vi "find nearest neighbors index float.vi"(0 "index_id":u64, 1 "nn":i32=1, 3 "Overwrite Lib Path":path, 5 "testset":sgl[][](array[numeric]), 9 "flann_params":T1 {"algorithm" items=["FLANN_INDEX_LINEAR"=0, "FLANN_INDEX_KDTREE"=1, "FLANN_INDEX_KMEANS"=2, "FLANN_INDEX_COMPOSITE"=3, "FLANN_INDEX_KDTREE_SINGLE"=4, "FLANN_INDEX_HIERARCHICAL"=5, "FLANN_INDEX_LSH"=6, "FLANN_INDEX_SAVED"=254, "FLANN_INDEX_AUTOTUNED"=255]; "centers_init" items=["FLANN_CENTERS_RANDOM", "FLANN_CENTERS_GONZALES", "FLANN_CENTERS_KMEANSPP", "FLANN_CENTERS_GROUPWISE"]; "log_level" items=["FLANN_LOG_NONE", "FLANN_LOG_FATAL", "FLANN_LOG_ERROR", "FLANN_LOG_WARN", "FLANN_LOG_INFO", "FLANN_LOG_DEBUG"]}, 11 "error in (no error)":errorcluster) -> (4 "index_id out":u64, 6 "Indices":i32[][](array[numeric]), 8 "Dists":sgl[][](array[numeric]), 10 "flann_params":T1 {"algorithm" items=["FLANN_INDEX_LINEAR"=0, "FLANN_INDEX_KDTREE"=1, "FLANN_INDEX_KMEANS"=2, "FLANN_INDEX_COMPOSITE"=3, "FLANN_INDEX_KDTREE_SINGLE"=4, "FLANN_INDEX_HIERARCHICAL"=5, "FLANN_INDEX_LSH"=6, "FLANN_INDEX_SAVED"=254, "FLANN_INDEX_AUTOTUNED"=255]; "centers_init" items=["FLANN_CENTERS_RANDOM", "FLANN_CENTERS_GONZALES", "FLANN_CENTERS_KMEANSPP", "FLANN_CENTERS_GROUPWISE"]; "log_level" items=["FLANN_LOG_NONE", "FLANN_LOG_FATAL", "FLANN_LOG_ERROR", "FLANN_LOG_WARN", "FLANN_LOG_INFO", "FLANN_LOG_DEBUG"]}, 15 "error out":errorcluster)   [LabVIEW 2020, in "KD Tree.lvlib"]
doc: "FLANN_EXPORT int flann_find_nearest_neighbors_index_double(flann_index_t index_id,\n double* testset,\n int trows,\n int* indices,\n double* dists,\n int nn,\n struct FLANNParameters* flann_params);"
uses:
  KD Tree.lvlib
  Flann Params.ctl
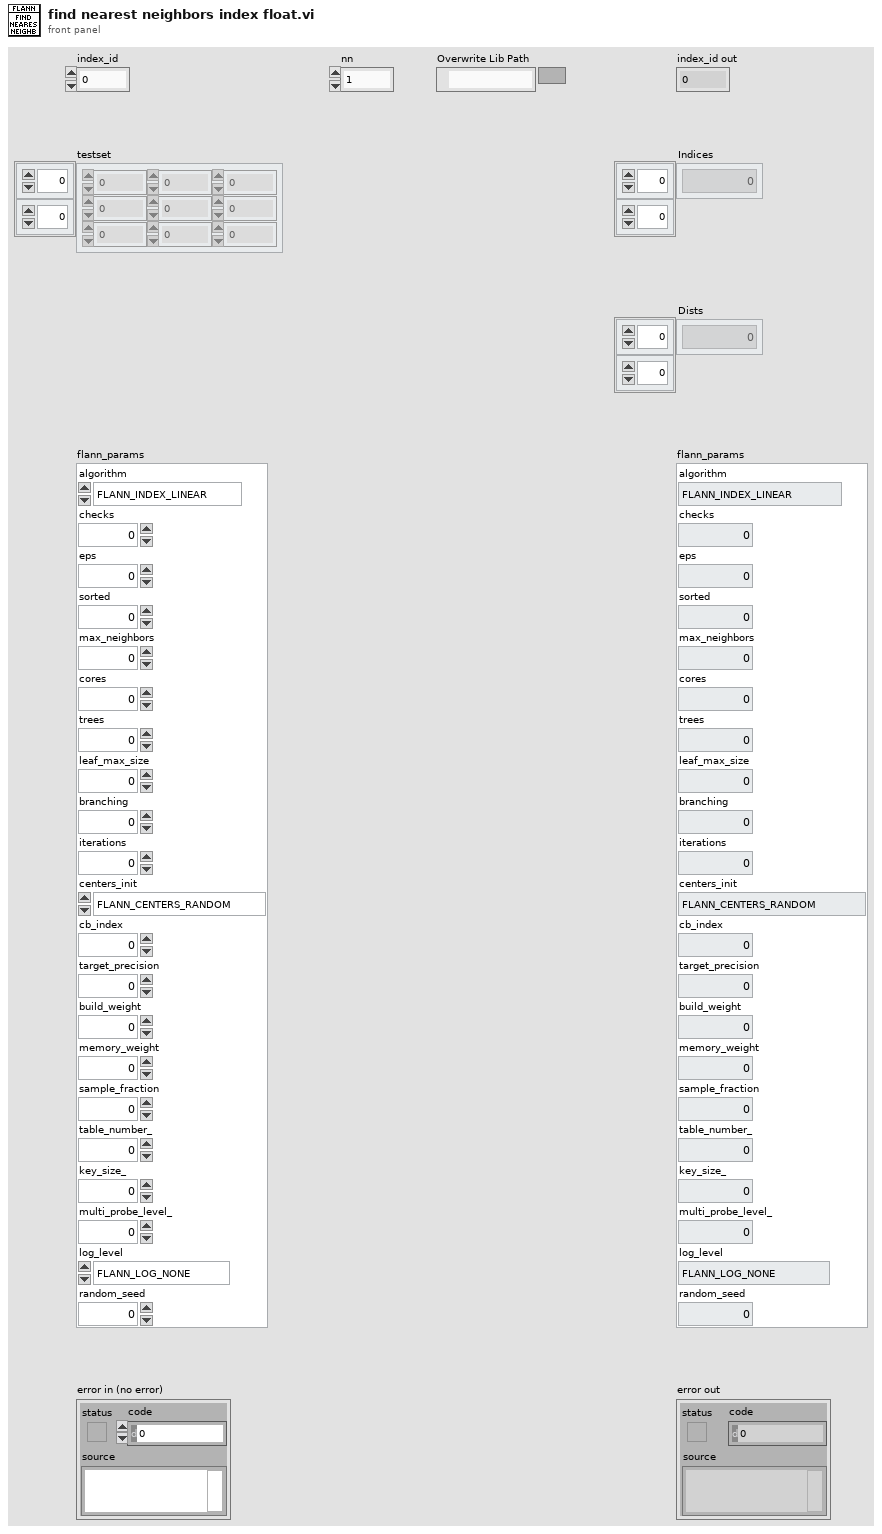
[diagram p1: front panel]
types:
  T1 = typedef "KD Tree.lvlib/Flann Params.ctl" = cluster{"algorithm":u32, "checks":i32, "eps":sgl, "sorted":i32, "max_neighbors":i32, "cores":i32, "trees":i32, "leaf_max_size":i32, "branching":i32, "iterations":i32, "centers_init":u32, "cb_index":sgl, "target_precision":sgl, "build_weight":sgl, "memory_weight":sgl, "sample_fraction":sgl, "table_number_":u32, "key_size_":u32, "multi_probe_level_":u32, "log_level":u32, "random_seed":i32}
  T2 = typedef "Semaphore RefNum" = refnum<k1>
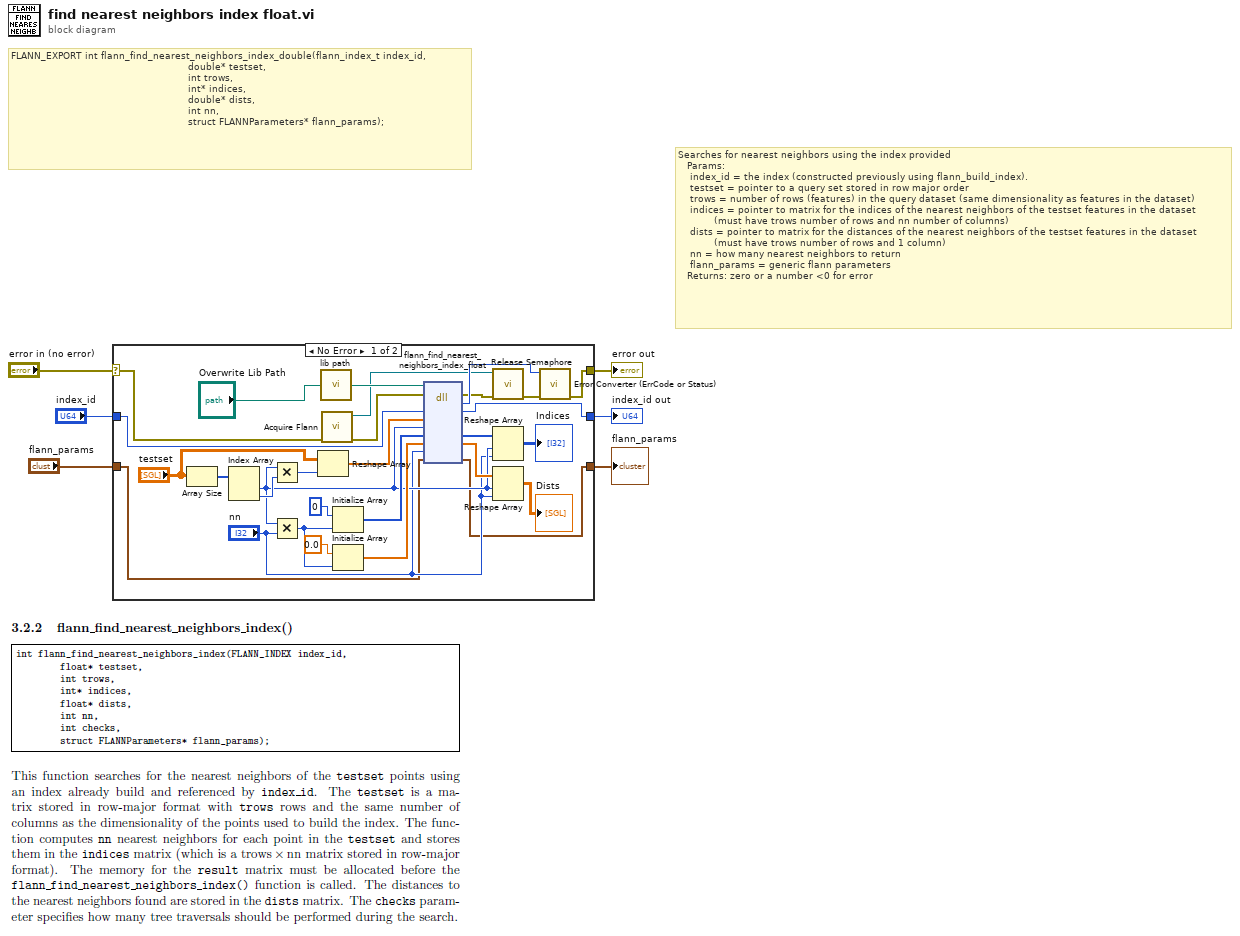
[diagram p0: block diagram]
diagram:
  # "Searches for nearest neighbors using the index provided\n   Params:\n    index_id = the index (constructed previously using flann_build_index).\n    testset = pointer to a query set stored in row major order\n    trows = number of rows (features) in the query dataset (same dimensionality as features in the dataset)\n    indices = pointer to matrix for the indices of the nearest neighbors of the testset features in the dataset\n            (must have trows number of rows and nn number of columns)\n    dists = pointer to matrix for the distances of the nearest neighbors of the testset features in the dataset\n            (must have trows number of rows and 1 column)\n    nn = how many nearest neighbors to return\n    flann_params = generic flann parameters\n   Returns: zero or a number <0 for error"
  # "FLANN_EXPORT int flann_find_nearest_neighbors_index_double(flann_index_t index_id,\n                                                           double* testset,\n                                                           int trows,\n                                                           int* indices,\n                                                           double* dists,\n                                                           int nn,\n                                                           struct FLANNParameters* flann_params);"
  n1 = case shown="No Error" "error in (no error)" {
    selector: "error in (no error)" -> [w16 w38]
    tunnel: [w17 w38] -> w6
    tunnel: "index_id" -> [w15 w37]
    tunnel: [w14 w37] -> w3
    tunnel: "flann_params" -> [w13 w36]
    tunnel: [w12 w36] -> w1
    frame No Error {
      n2 = Array Size(array="testset") -> (size(s)=w33:i32[])
      n3 = Index Array(array=w33) -> (element #1=w20:i32, element #2=w31:i32)  [unwired: 2 in]
      n4 = Multiply(x=w20, y=w31) -> (x*y=w30:i32)
      n5 = Multiply(x=w20, y="nn") -> (x*y=w26:i32)
      n6 = Reshape Array("testset", w30) -> (w29:sgl[])
      n7 = call "lib path.vi"("Overwrite Lib Path"="Overwrite Lib Path") -> ("lib path"=w11:path)
      n8 = call "Acquire Flann.vi"("error in (no error)"=w16) -> ("error out"=w9:errorcluster, "semaphore"=w7:T2)  [unwired: 9 in]
      n9 = Initialize Array(0, w26) -> (w27:i32[])
      n10 = Initialize Array(0.0, w26) -> (w24:dbl[])
      n11 = dll-call lib="E:/Labview/LV 2020/Libs/flann/flann.dll" fn="flann_find_nearest_neighbors_index_float"(path in=w11, error in=w9, "index_id"=w15, "testset"=w29, "trows"=w20, "indices"=w27, "dists"=w24, "nn"="nn", "flann_params"=w13) -> (error out=w34:errorcluster, "return type"=w35:i32, "index_id"=w14:u64, "indices"=w23:i32[], "dists"=w21:sgl[], "flann_params"=w12:T1)  [unwired: 4 in, 1 out]
      n12 = call <vilib>:"Release Semaphore.vi"("error in (no error)"=w34, "semaphore"=w7) -> ("error out"=w8:errorcluster)  [unwired: 4 in, 1 out]
      n13 = Reshape Array(w23, w20, "nn") -> (→"Indices":i32[][])
      n14 = Reshape Array(w21, w20, "nn") -> (→"Dists":sgl[][])
      n15 = call "Error Converter (ErrCode or Status).vi"("error in (no error)"=w8, "error code"=w35) -> ("error out"=w17:errorcluster)  [unwired: 9 in]
    }
    frame Error {
    }
  }
  "error out" <- w6
  "index_id out" <- w3
  "flann_params" <- w1
